vi "Practica_30.vi"() -> ()   [LabVIEW 2019]
panel:
  in  "Cyan Button":bool
  in  "Amarillo Button":bool
  in  "Magenta Button":bool
  out "Cyan":dbl(slide) scale=0.0..100.0
  out "Amarillo":dbl(slide) scale=0.0..100.0
  out "Magenta":dbl(slide) scale=0.0..100.0
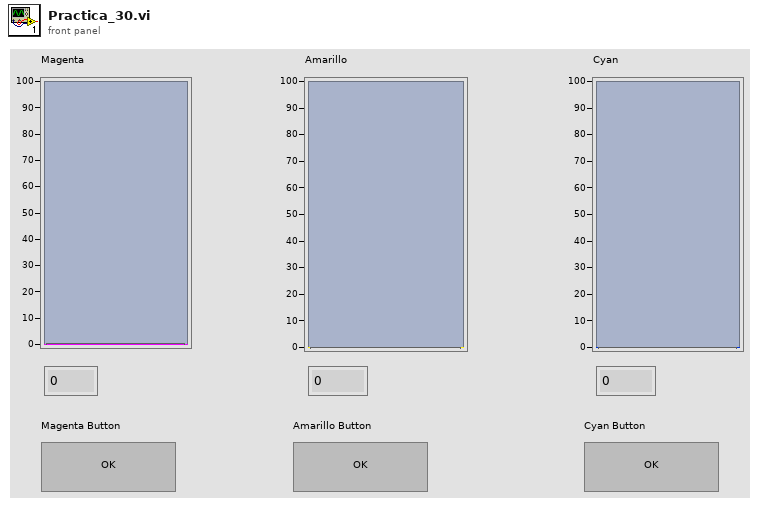
[diagram p1: front panel]
types:
  T1 = enum16{"Inicio", "vacia magenta", "Vacia amarillo", "Vacia cyan", "a", "b", "c", "d", "e", "f", "g", "h"}
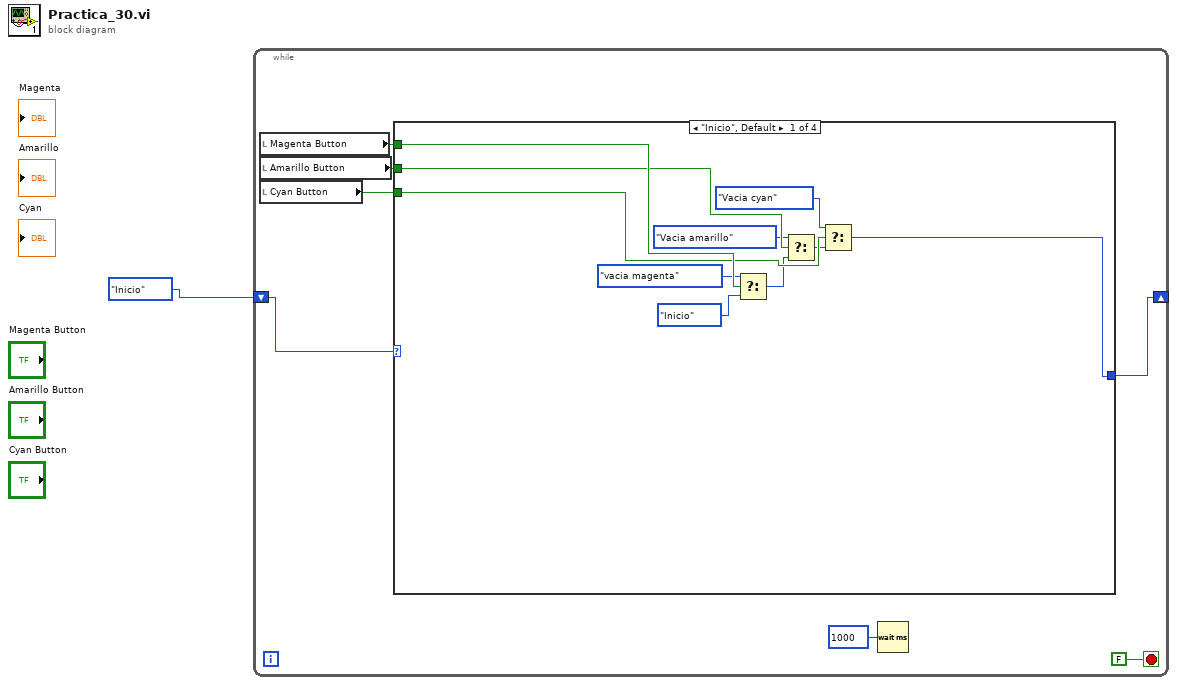
[diagram p0: block diagram]
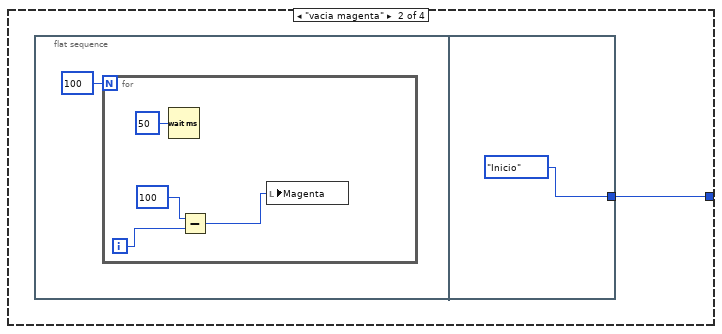
[diagram p2: hidden frame]
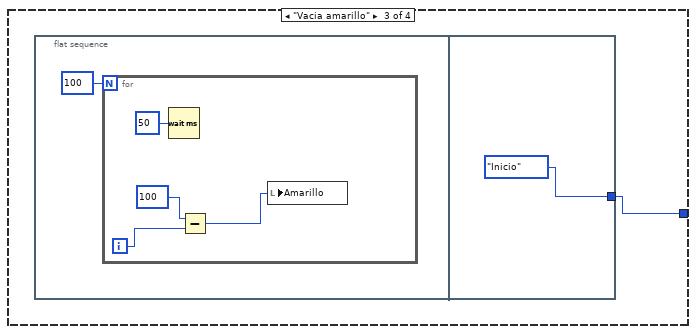
[diagram p3: hidden frame]
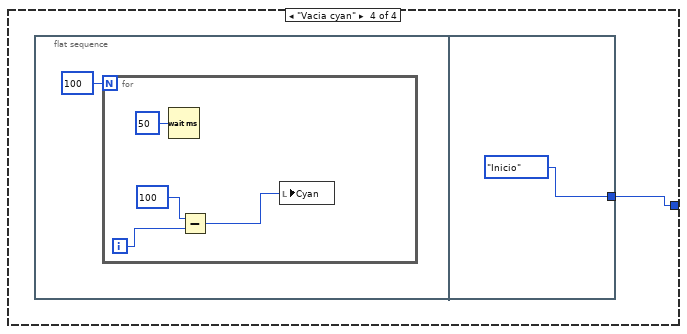
[diagram p4: hidden frame]
diagram:
  n1 = while {
    shift-right: [w2] -> _
    shift-left: T1."Inicio" -> [w6]
    stop <- FALSE stop-if-true
    n2 = local read "Magenta Button"() -> (w5:bool)
    n3 = local read "Amarillo Button"() -> (w4:bool)
    n4 = local read "Cyan Button"() -> (w3:bool)
    n5 = case shown="\"Inicio\", Default" w6 {
      tunnel: w5 -> [w18 _ _ _]
      tunnel: w4 -> [w15 _ _ _]
      tunnel: w3 -> [w13 _ _ _]
      tunnel: [w9 w19 w26 w33] -> w2
      frame "Inicio", Default {
        n6 = Select(t=T1."vacia magenta", s=w18, f=T1."Inicio") -> (s? t:f=w11:T1)
        n7 = Select(t=T1."Vacia amarillo", s=w15, f=w11) -> (s? t:f=w10:T1)
        n8 = Select(t=T1."Vacia cyan", s=w13, f=w10) -> (s? t:f=w9:T1)
      }
      frame "vacia magenta" {
        n9 = flat-sequence {
          tunnel: [T1."Inicio"] -> w19
          frame #0 {
            n10 = for {
              N: 100 -> [_]
              i -> [w23]
              n11 = Wait (ms)(milliseconds to wait=u32 50) -> ()  [unwired: 1 out]
              n12 = Subtract(x=100, y=w23) -> (x-y=w22:i32)
              n13 = local write "Magenta"(w22) -> ()
            }
          }
          frame #1 {
          }
        }
      }
      frame "Vacia amarillo" {
        n14 = flat-sequence {
          tunnel: [T1."Inicio"] -> w26
          frame #0 {
            n15 = for {
              N: 100 -> [_]
              i -> [w30]
              n16 = Wait (ms)(milliseconds to wait=u32 50) -> ()  [unwired: 1 out]
              n17 = Subtract(x=100, y=w30) -> (x-y=w29:i32)
              n18 = local write "Amarillo"(w29) -> ()
            }
          }
          frame #1 {
          }
        }
      }
      frame "Vacia cyan" {
        n19 = flat-sequence {
          tunnel: [T1."Inicio"] -> w33
          frame #0 {
            n20 = for {
              N: 100 -> [_]
              i -> [w37]
              n21 = Wait (ms)(milliseconds to wait=u32 50) -> ()  [unwired: 1 out]
              n22 = Subtract(x=100, y=w37) -> (x-y=w36:i32)
              n23 = local write "Cyan"(w36) -> ()
            }
          }
          frame #1 {
          }
        }
      }
    }
    n24 = Wait (ms)(milliseconds to wait=u32 1000) -> ()  [unwired: 1 out]
  }
